vi "Array - Failure Message.vi"() -> ()   [LabVIEW 2017, in "Transparent Assertions.Tests.lvlib" / "Assert Collection Equivalent.lvlib"]
uses:
  Assert Collection Equivalent.lvlib
  src/Transparent Assertions/Transparent Assertions.lvlib
panel:
  out "error out":errorcluster
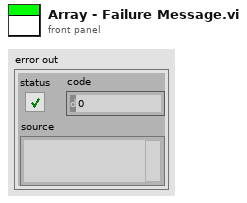
[diagram p1: front panel]
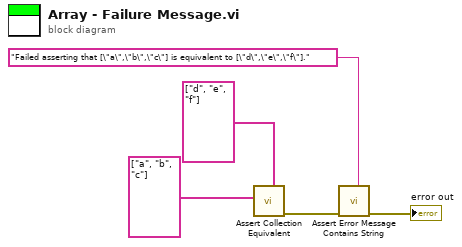
[diagram p0: block diagram]
diagram:
  n1 = call "Assert Collection Equivalent.vi"("Expected"=string[] ["d", "e", "f"], "Collection"=string[] ["a", "b", "c"]) -> ("error out"=w3:errorcluster)  [unwired: 9 in]
  n2 = call "Assert Error Message Contains String.vi"("Expected"="Failed asserting that [\"a\",\"b\",\"c\"] is equivalent to [\"d\",\"e\",\"f\"].", "error in (no error)"=w3) -> ("error out"=→"error out":errorcluster)  [unwired: 9 in]
